vi "Database Test Null.vi"() -> ()   [LabVIEW 2013]
doc: "This exmaple demonstrates how to verify whether a variant in the database is Null or not. This example first inserts two Null values and some numeric and string values to the database. This example then uses the Database Variant To Data function to display these values and uses the DB Tools Null VI to verify whether the value is Null or not. \n\nComplete the following steps to use this example VI:\n1. Select <B>INSERT</B> from the <B>Action</B> pull-down menu.\n2. Run this VI to insert values to the database.\n3. Select <B>READ</B> from the <B>Action</B> pull-down menu.\n4. Run this VI again to read the inserted values.\n\nThe <B>Value</B> array displays the data read from the database. The <B>Value is Null</B> array displays whether the corresponding data in <B>Value</B> is a Null value or not."
uses:
  Auxilliary.llb/DB Tools Column Info.ctl
  Auxilliary.llb/DB Tools DataTypes.ctl
  Auxilliary.llb/DB Tools Parameter Info.ctl
  Auxilliary.llb/DB Tools Parameter Dir.ctl
  Connection.llb/DB Tools Open Connec (Path).vi
  Command.llb/Cmd Set Parameter Value (C).vi
  Command.llb/Cmd Execute.vi
  Recordset.llb/Rec Destroy - Command.vi
  Command.llb/Cmd Delete.vi
  Connection.llb/Conn Execute.vi
  Recordset.llb/Rec Destroy - Connection.vi
  _DB Variant To Data/Database Variant To Data.xnode
  NI_Database_API_64.lvlib
panel:
  in  "parameters":T1[](array[typedef])=[{"parameter name"="Str", "type"=enum."String", "direction"=enum."Input", "value"=variant}, {"parameter name"="DT", "type"=enum."Date/Time", "direction"=enum."Input", "value"=variant}, {"parameter name"="DBL", "type"=enum."Double (DBL)", "direction"=enum."Input", "value"=variant}, {"parameter name"="I32", "type"=enum."Long (I32)", "direction"=enum."Input", "value"=variant}]
  in  "column information":T4[](array[typedef])=[{"column name"="Str", "data type"=enum."String", "size"=32, "allow null?"=TRUE}, {"column name"="DT", "data type"=enum."Date/Time", "size"=0, "allow null?"=TRUE}, {"column name"="DBL", "data type"=enum."Double (DBL)", "size"=0, "allow null?"=TRUE}, {"column name"="I32", "data type"=enum."Long (I32)", "size"=0, "allow null?"=TRUE}]
  out "error out":errorcluster
  out "Value is NULL?":bool[][](array[boolean])
  out "Value":string[][](array[string])
  in  "Action":enum16{"INSERT", "READ"}(ring)
  # "INSTRUCTIONS:\n\nThis exmaple demonstrates how to verify whether a variant in the database is Null or not. This example first inserts two Null values and some numeric and string values to the database. This example then uses the Database Variant To Data function to display these values and uses the DB Tools Null VI to verify whether the value is Null or not. \n\nComplete the following steps to use this example VI:\n1. Select INSERT from the Action pull-down menu.\n2. Run this VI to insert values to the database.\n3. Select READ from the Action pull-down menu.\n4. Run this VI again to read the inserted values.\n\nThe Value array displays the data read from the database. The Value is Null array displays whether the corresponding data in Value is a Null value or not."
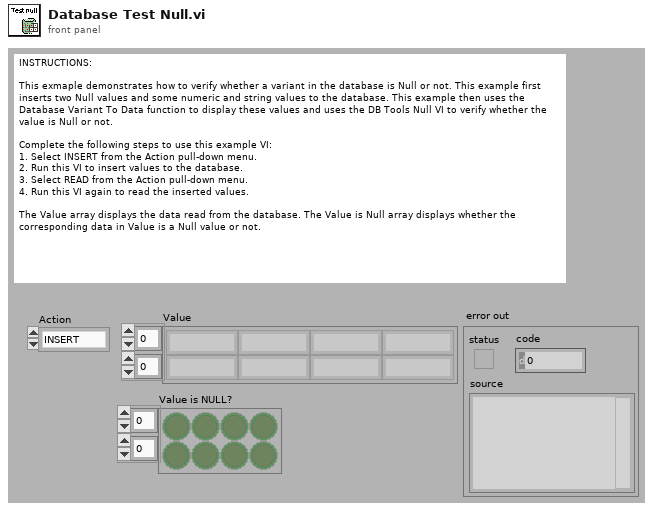
[diagram p1: front panel]
types:
  T1 = typedef "NI_Database_API_64.lvlib/DB Tools Parameter Info.ctl" = cluster{"parameter name":string, "type":T2, "direction":T3, "value":variant}
  T2 = typedef "NI_Database_API_64.lvlib/DB Tools DataTypes.ctl" = enum16{"String", "Long (I32)", "Single (SGL)", "Double (DBL)", "Date/Time", "Binary"}
  T3 = typedef "NI_Database_API_64.lvlib/DB Tools Parameter Dir.ctl" = enum32{"Input", "Output", "Input/Output", "Return Value"}
  T4 = typedef "NI_Database_API_64.lvlib/DB Tools Column Info.ctl" = cluster{"column name":string, "data type":T2, "size":i32, "allow null?":bool}
  T5 = typedef "NI_Database_API_64.lvlib/Conn ObjectReference.ctl" = refnum<k1>
  T6 = typedef "NI_Database_API_64.lvlib/Cmd ObjectReference.ctl" = refnum<k1>
  T7 = typedef "NI_Database_API_64.lvlib/Cmd-Rec Object Reference.ctl" = refnum<k1>
  T8 = typedef "NI_Database_API_64.lvlib/Rec ObjectReference.ctl" = refnum<k1>
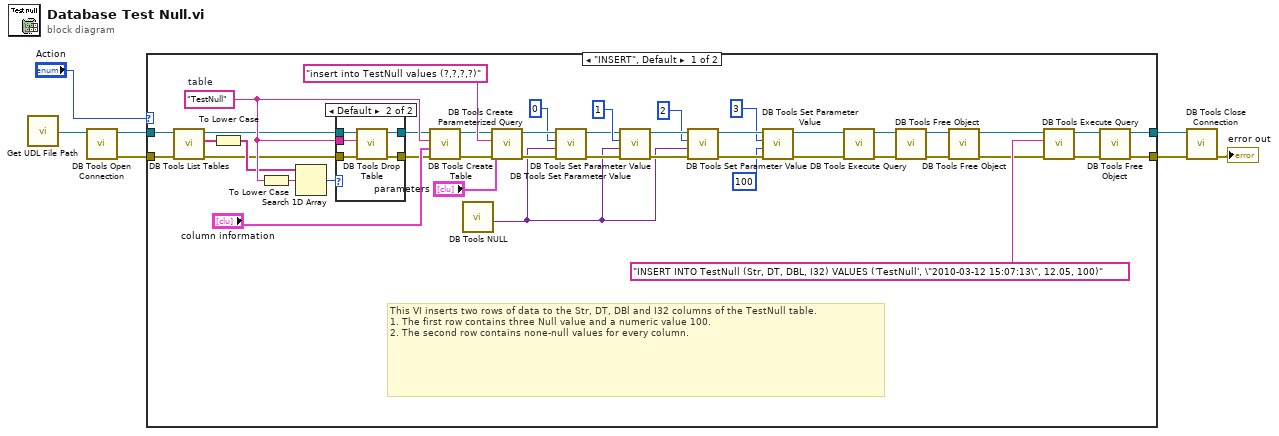
[diagram p0: block diagram]
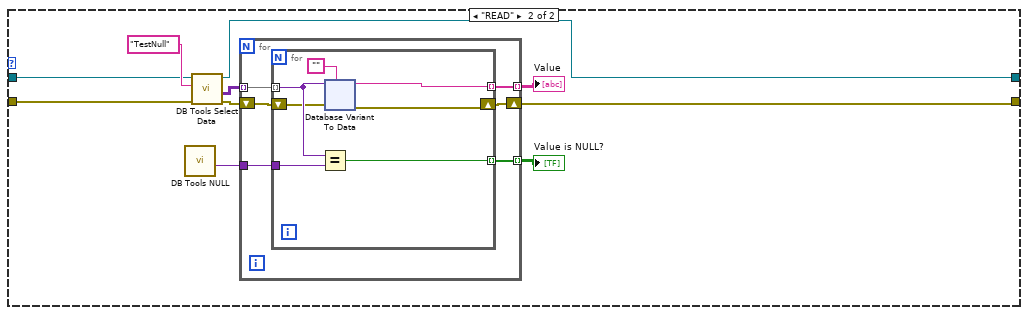
[diagram p3: hidden frame]
diagram:
  n1 = call "Get UDL File Path.vi"() -> ("UDL file path"=w1:path)  [unwired: 1 in]
  n2 = call-poly "DB Tools Open Connection.vi"("connection information"=w1) -> ("error out"=w3:errorcluster, "connection reference"=w4:T5)  [unwired: 7 in]
  n3 = case shown="\"INSERT\", Default" "Action" {
    tunnel: w4 -> [w20 w59]
    tunnel: w3 -> [w19 w65]
    tunnel: [w47 w61] -> w6
    tunnel: [w46 w58] -> w5
    frame "INSERT", Default {
      w31 = "TestNull"  # table
      # "This VI inserts two rows of data to the Str, DT, DBl and I32 columns of the TestNull table. \n1. The first row contains three Null value and a numeric value 100. \n2. The second row contains none-null values for every column."
      n4 = call "DB Tools List Tables.vi"("error in (no error)"=w19, "connection reference"=w20) -> ("error out"=w24:errorcluster, "tables"=w23:string[], "connection reference out"=w25:T5)  [unwired: 3 in]
      n5 = To Lower Case(string=w23) -> (all lower case string=w26:string[])
      n6 = To Lower Case(string=w31) -> (all lower case string=w27:string)
      n7 = Search 1D Array(1D array=w26, element=w27) -> (index of element=w28:i32)  [unwired: 1 in]
      n8 = case shown="Default" w28 {
        tunnel: w24 -> [w51 w57]
        tunnel: w25 -> [w52 w56]
        tunnel: [w52 w55] -> w30
        tunnel: [w51 w54] -> w29
        tunnel: w31 -> [_ w53]
        frame -1 {
        }
        frame Default {
          n9 = call "DB Tools Drop Table.vi"("error in (no error)"=w57, "table"=w53, "connection reference"=w56) -> ("error out"=w54:errorcluster, "connection reference out"=w55:T5)  [unwired: 5 in]
        }
      }
      n10 = call "DB Tools Create Table.vi"("error in (no error)"=w29, "column information"="column information", "table"=w31, "connection reference"=w30) -> ("error out"=w39:errorcluster, "connection reference out"=w32:T5)  [unwired: 4 in]
      n11 = call "DB Tools NULL.vi"() -> ("NULL"=w8:variant)  [unwired: 10 in, 1 out]
      n12 = call "DB Tools Create Parameterized Query.vi"("error in (no error)"=w39, "parameters"="parameters", "SQL query"="insert into TestNull values (?,?,?,?)", "connection reference"=w32) -> ("error out"=w42:errorcluster, "command reference"=w43:T6)  [unwired: 2 in, 2 out]
      n13 = call-poly "DB Tools Set Parameter Value.vi"("error in (no error)"=w42, "value"=w8, "parameter index"=0, "command reference"=w43) -> ("error out"=w34:errorcluster, "command reference out"=w35:T6)  [unwired: 4 out]
      n14 = call-poly "DB Tools Set Parameter Value.vi"("error in (no error)"=w34, "value"=w8, "parameter index"=1, "command reference"=w35) -> ("error out"=w14:errorcluster, "command reference out"=w13:T6)  [unwired: 4 out]
      n15 = call-poly "DB Tools Set Parameter Value.vi"("error in (no error)"=w14, "value"=w8, "parameter index"=2, "command reference"=w13) -> ("error out"=w15:errorcluster, "command reference out"=w16:T6)  [unwired: 4 out]
      n16 = call-poly "DB Tools Set Parameter Value.vi"("error in (no error)"=w15, "value"=100, "parameter index"=3, "command reference"=w16) -> ("error out"=w18:errorcluster, "command reference out"=w17:T6)  [unwired: 4 out]
      n17 = call-poly "DB Tools Execute Query.vi"("error in (no error)"=w18, "command reference"=w17) -> ("error out"=w36:errorcluster, "command-recordset reference"=w37:T7)  [unwired: 2 in, 4 out]
      n18 = call-poly "DB Tools Free Object.vi"("error in (no error)"=w36, "command-recordset reference"=w37) -> ("error out"=w38:errorcluster, "command reference"=w45:T6)  [unwired: 8 out]
      n19 = call-poly "DB Tools Free Object.vi"("error in (no error)"=w38, "command reference"=w45) -> ("error out"=w21:errorcluster, "connection reference"=w22:T5)  [unwired: 8 out]
      n20 = call-poly "DB Tools Execute Query.vi"("error in (no error)"=w21, "SQL query"="INSERT INTO TestNull (Str, DT, DBL, I32) VALUES ('TestNull', \"2010-03-12 15:07:13\", 12.05, 100)", "connection reference"=w22) -> ("error out"=w49:errorcluster, "recordset reference"=w48:T8)  [unwired: 1 in, 4 out]
      n21 = call-poly "DB Tools Free Object.vi"("error in (no error)"=w49, "recordset reference"=w48) -> ("error out"=w47:errorcluster, "connection reference"=w46:T5)  [unwired: 8 out]
    }
    frame "READ" {
      n22 = call "DB Tools NULL.vi"() -> ("NULL"=w60:variant)  [unwired: 10 in, 1 out]
      n23 = call "DB Tools Select Data.vi"("error in (no error)"=w65, "table"="TestNull", "connection reference"=w59) -> ("error out"=w62:errorcluster, "data"=w67:variant[][], "connection reference out"=w58:T5)  [unwired: 1 in, 2 out]
      n24 = for {
        tunnel: w67 -> [w73] mode=indexing
        tunnel: [w72] -> w66 mode=indexing
        tunnel: [w71] -> w64 mode=indexing
        shift-right: [w69] -> w61
        shift-left: w62 -> [w70]
        tunnel: w60 -> [w68]
        n25 = for {
          tunnel: w73 -> [w76] mode=indexing
          tunnel: [w79] -> w72 mode=indexing
          tunnel: [w78] -> w71 mode=indexing
          shift-right: [w74] -> w69
          shift-left: w70 -> [w75]
          tunnel: w68 -> [w77]
          n26 = Equal?(x=w76, y=w77) -> (x = y?=w78:bool)
          n27 = xnode "Database Variant To Data"("database variant"=w76, "error in"=w75, "type"="") -> ("data"=w79:string, "error out"=w74:errorcluster)
        }
      }
      "Value" <- w66
      "Value is NULL?" <- w64
    }
  }
  n28 = call "DB Tools Close Connection.vi"("error in (no error)"=w6, "connection reference"=w5) -> ("error out"=→"error out":errorcluster)  [unwired: 5 out]
